vi "Main.vi"(8 "error in":errorcluster, 11 "Main UI in":refnum<class "Main UI.lvclass">) -> (0 "error out":errorcluster, 3 "Main UI out":refnum<class "Main UI.lvclass">)   [LabVIEW 2017, in "Main UI.lvclass"]
doc: "The <b>Queued Message Handler</b> of the Worker that owns this VI."
uses:
  Main UI.lvclass
  C:/Program Files (x86)/National Instruments/LabVIEW 2017/vi.lib/addons/_Workers/Library/Classes/Worker/Worker.lvclass
  Initialization Data.ctl
  Response Cases.ctl
  Main UI.lvclass/Main UI.ctl
  subPanel Worker/subPanel Worker.lvclass
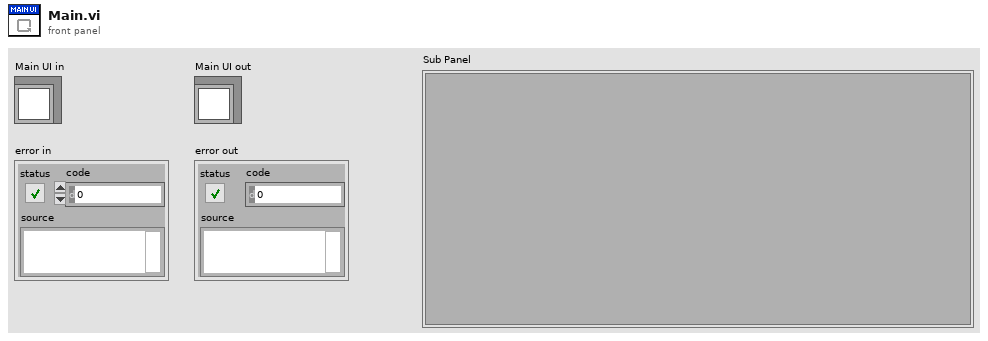
[diagram p1: front panel]
types:
  T1 = typedef "Main UI.lvclass/Initialization Data.ctl" = cluster{"Response Cases":T2}
  T2 = typedef "Main UI.lvclass/Response Cases.ctl" = cluster{"Placeholder - Can be deleted":string}
  T3 = typedef "subPanel Worker.lvclass/rwr_Get Main VI Ref Reply.ctl" = cluster{"VI Ref":refnum<vi>}
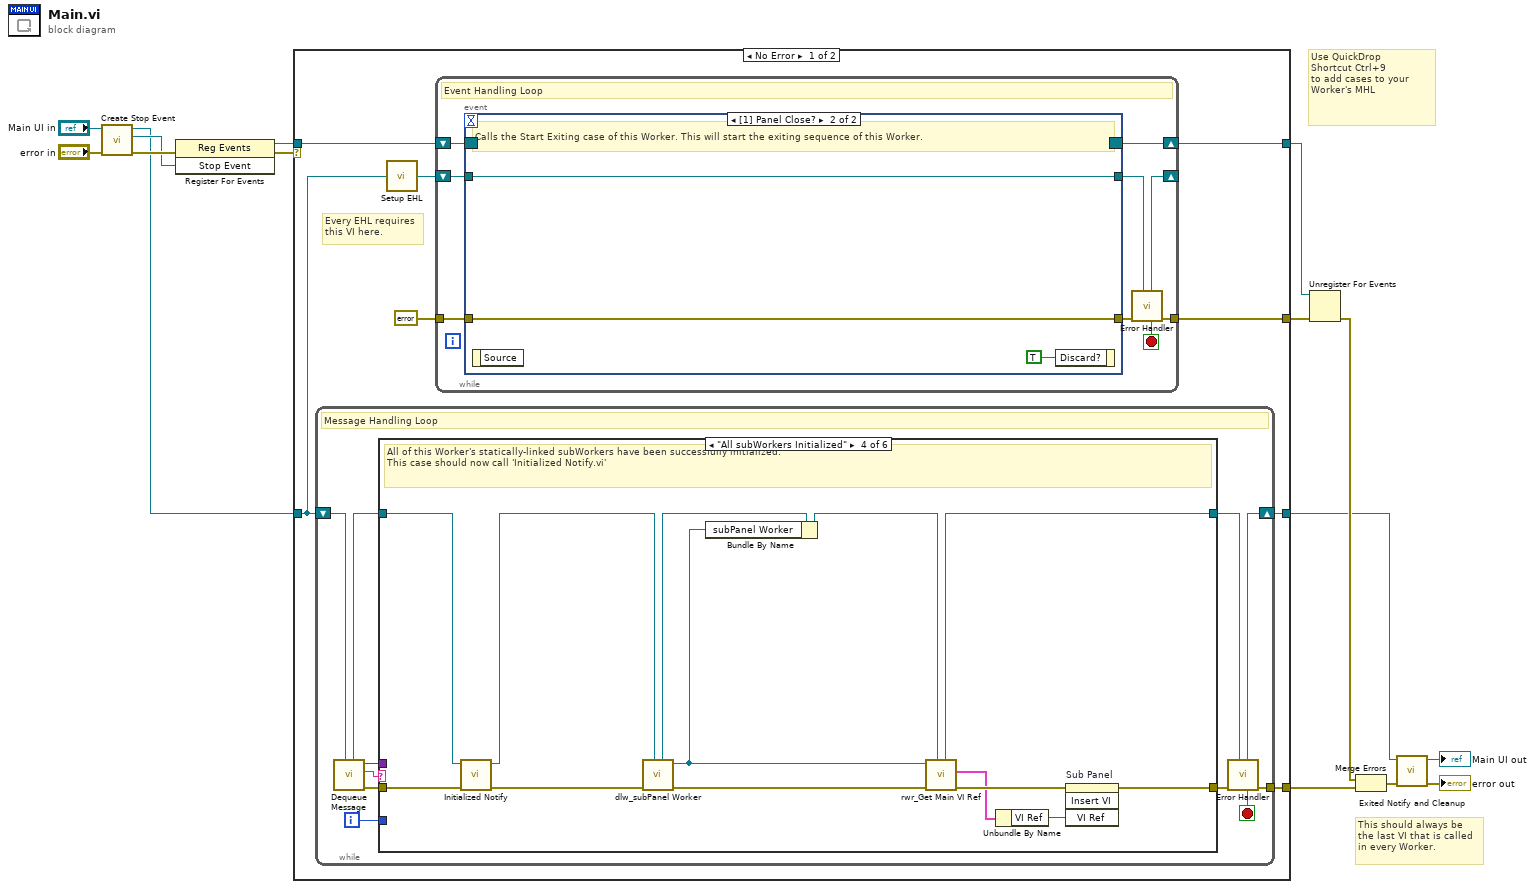
[diagram p0: block diagram]
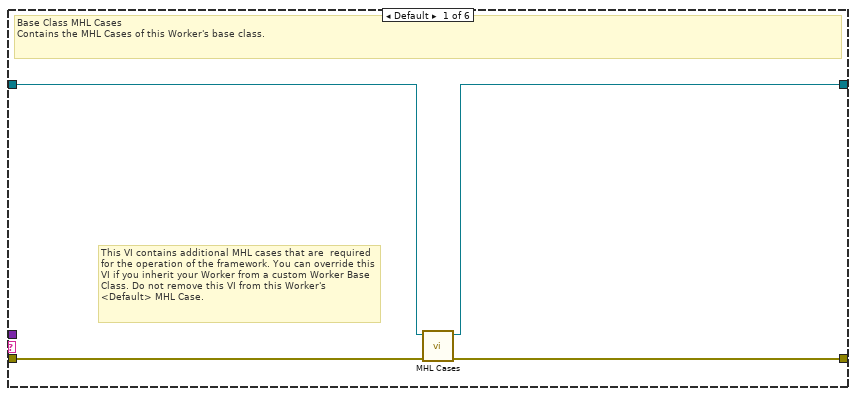
[diagram p2: hidden frame]
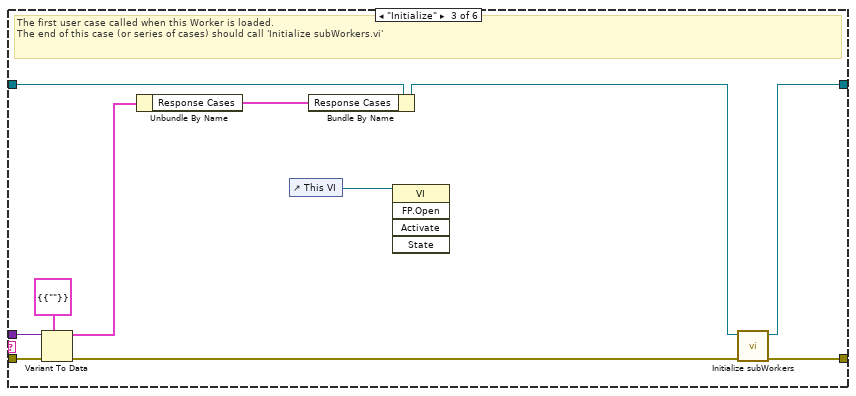
[diagram p4: hidden frame]
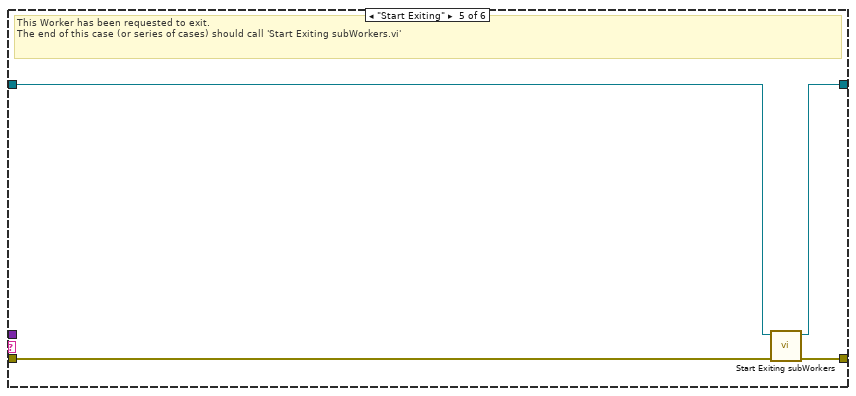
[diagram p5: hidden frame]
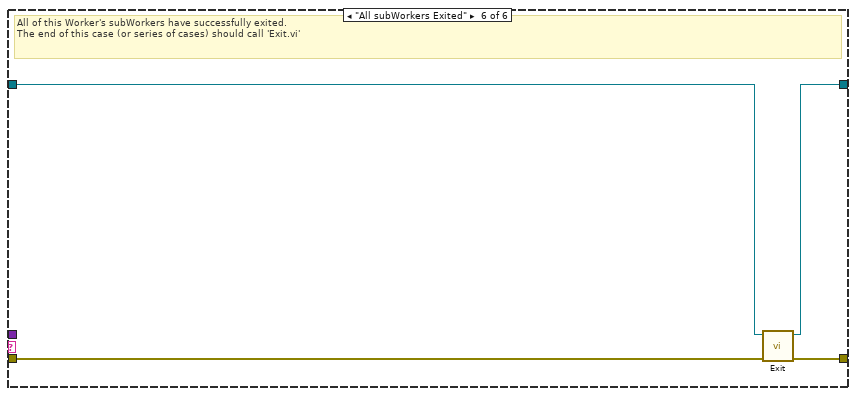
[diagram p6: hidden frame]
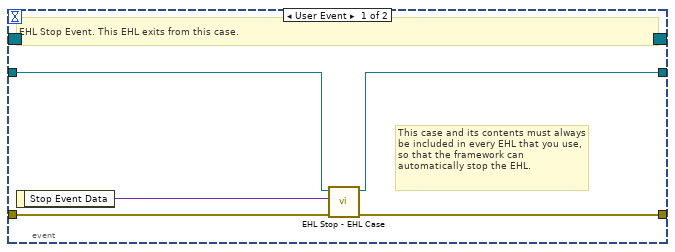
[diagram p7: hidden frame]
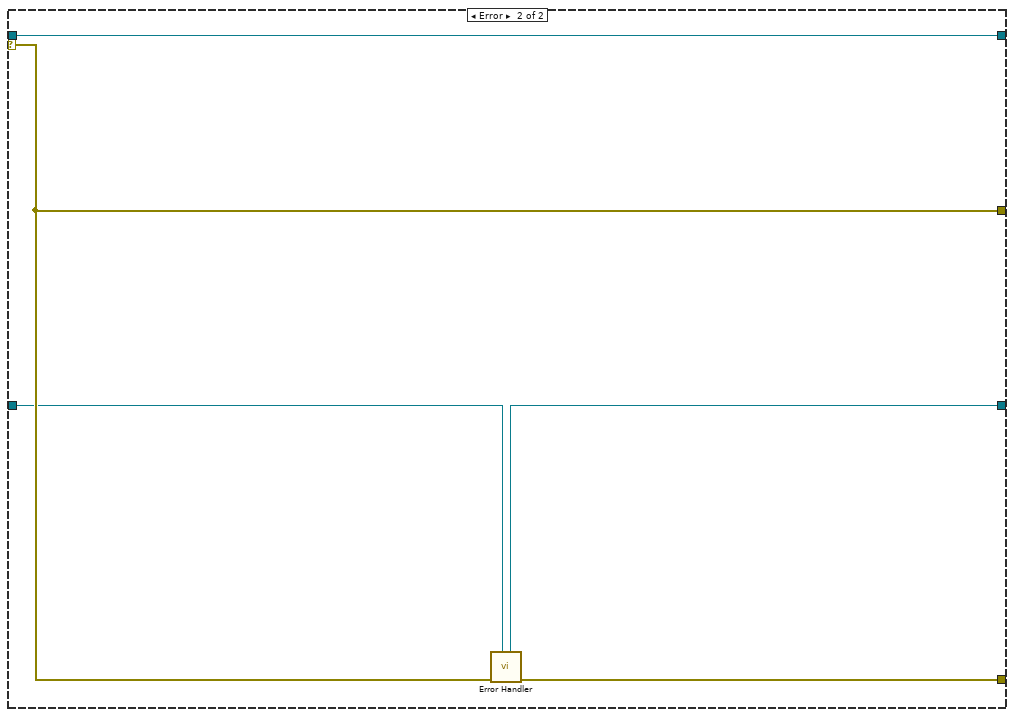
[diagram p8: hidden frame]
diagram:
  # "Use QuickDrop\nShortcut Ctrl+9\nto add cases to your\nWorker's MHL"
  # "This should always be the last VI that is called in every Worker."
  n1 = call-dynamic "Create Stop Event.vi"("error in"="error in", "Worker"="Main UI in") -> ("error out"=w10:errorcluster, "Stop Event"=w7:refnum<user-event>, "Worker out"=w4:refnum<class "Main UI.lvclass">)  [unwired: 7 in]
  n2 = register-events(error in=w10, w7) -> (reference out=w9:refnum<event-registration>, error out=w1:errorcluster)  [unwired: 1 in]
  n3 = case shown="No Error" w1 {
    tunnel: w4 -> [w18 w91]
    tunnel: [w16 w92] -> w8
    tunnel: w9 -> [w23 w93]
    tunnel: [w20 w94] -> w14
    tunnel: [w22 w93] -> w13
    tunnel: [w17 w90] -> w11
    selector: w1 -> [_ w94]
    frame No Error {
      # "Every EHL requires\nthis VI here."
      n4 = while {
        shift-right: [w32] -> w17
        shift-left: w18 -> [w34]
        tunnel: [w33] -> w16
        i -> [w24]
        stop <- w25 stop-if-true
        # "Message Handling Loop"
        n5 = call-dynamic "Dequeue Message.vi"("Worker"=w34) -> ("error out"=w31:errorcluster, "Case out"=w26:string, "Data out"=w27:variant, "Worker out"=w29:refnum<class "Main UI.lvclass">)  [unwired: 6 in, 1 out]
        n6 = case "Worker MHL Case Structure (DO NOT CHANGE LABEL NAME)" shown="\"All subWorkers Initialized\"" w26 {
          tunnel: w31 -> [w38 w39 w49 w63 w65 w72]
          tunnel: [w37 w39 w51 w55 w68 w71] -> w30
          tunnel: w29 -> [w36 w40 w48 w64 w66 w70]
          tunnel: [w35 w40 w50 w57 w67 w69] -> w28
          tunnel: w27 -> [_ _ w46 _ _ _]
          tunnel: w24 -> [_ _ _ _ _ _]
          frame Default {
            # "This VI contains additional MHL cases that are  required for the operation of the framework. You can override this VI if you inherit your Worker from a custom Worker Base Class. Do not remove this VI from this Worker's <Default> MHL Case."
            # "Base Class MHL Cases\nContains the MHL Cases of this Worker's base class."
            n7 = call-dynamic "MHL Cases.vi"("error in"=w38, "Worker in"=w36) -> ("error out"=w37:errorcluster, "Worker out"=w35:refnum<class "Main UI.lvclass">)  [unwired: 8 in]
          }
          frame "------------ FRAMEWORK CASES -----------" {
            # "Start of Workers Framework Cases"
          }
          frame "Initialize" {
            # "The first user case called when this Worker is loaded.\nThe end of this case (or series of cases) should call 'Initialize subWorkers.vi'"
            n8 = Variant To Data(error in=w49, type=T1 {"Response Cases"={"Placeholder - Can be deleted"=""}} ("Initialization Data"), Variant=w46) -> (data=w44:T1, error out=w47:errorcluster)
            n9 = Unbundle By Name(w44) -> ("Response Cases"=w43:T2)
            n10 = control-ref of="This VI"() -> (w41:refnum<vi>)
            n11 = Bundle By Name(cluster=w48, "Response Cases"=w43) -> (w45:refnum<class "Main UI.lvclass">)
            n12 = invoke class="VI" method="FP.Open"(reference=w41) -> ()  [unwired: 4 in, 5 out]
            n13 = call-dynamic "Initialize subWorkers.vi"("error in"=w47, "Worker"=w45) -> ("error out"=w51:errorcluster, "dup Worker out"=w50:refnum<class "Main UI.lvclass">)  [unwired: 8 in]
          }
          frame "All subWorkers Initialized" {
            # "All of this Worker's statically-linked subWorkers have been successfully initialized.\nThis case should now call 'Initialized Notify.vi'"
            n14 = call-dynamic "Initialized Notify.vi"("error in"=w63, "Worker"=w64) -> ("error out"=w62:errorcluster, "dup Worker out"=w60:refnum<class "Main UI.lvclass">)  [unwired: 8 in]
            n15 = call "dlw_subPanel Worker.vi"("Caller in"=w60, "error in"=w62) -> ("error out"=w61:errorcluster, "subPanel Worker out"=w52:refnum<class "subPanel Worker.lvclass">, "dup Caller out"=w59:refnum<class "Main UI.lvclass">)  [unwired: 7 in]
            n16 = Bundle By Name(cluster=w59, "subPanel Worker"=w52) -> (w58:refnum<class "Main UI.lvclass">)
            n17 = call "rwr_Get Main VI Ref.vi"("Caller in"=w58, "error in"=w61, "subPanel Worker in"=w52) -> ("error out"=w56:errorcluster, "Reply Data out"=w54:T3, "dup Caller out"=w57:refnum<class "Main UI.lvclass">)  [unwired: 5 in, 1 out]
            n18 = Unbundle By Name(w54) -> ("VI Ref"=w53:refnum<vi>)
            n19 = invoke on="Sub Panel" class="SubPnl" method="Insert VI"(error in=w56, "VI Ref"=w53) -> (error out=w55:errorcluster)  [unwired: 2 in, 3 out]
          }
          frame "Start Exiting" {
            # "This Worker has been requested to exit. \nThe end of this case (or series of cases) should call 'Start Exiting subWorkers.vi'"
            n20 = call-dynamic "Start Exiting subWorkers.vi"("error_in"=w65, "Worker"=w66) -> ("error out"=w68:errorcluster, "dup Worker out"=w67:refnum<class "Main UI.lvclass">)  [unwired: 8 in]
          }
          frame "All subWorkers Exited" {
            # "All of this Worker's subWorkers have successfully exited. \nThe end of this case (or series of cases) should call 'Exit.vi'"
            n21 = call-dynamic "Exit.vi"("error_in"=w72, "Worker"=w70) -> ("error out"=w71:errorcluster, "dup Worker out"=w69:refnum<class "Main UI.lvclass">)  [unwired: 8 in]
          }
        }
        n22 = call-dynamic "Error Handler.vi"("Worker"=w28, "error_in"=w30) -> ("error out"=w33:errorcluster, "Stop Loop"=w25:bool, "Worker out"=w32:refnum<class "Main UI.lvclass">)  [unwired: 7 in]
      }
      n23 = call-dynamic "Setup EHL.vi"("Worker"=w18) -> ("Worker out"=w19:refnum<class "Main UI.lvclass">)  [unwired: 14 in]
      n24 = while "Event Handling Loop" {
        shift-right: [w81] -> w22
        shift-left: w23 -> [w80]
        tunnel: [w76] -> w20
        tunnel: errorcluster {"status"=FALSE, "code"=0, "source"=""} ("error constant") -> [w78]
        shift-right: [w74] -> _
        shift-left: w19 -> [w79]
        stop <- w73 stop-if-true
        # "Event Handling Loop"
        n25 = event shown="[1] Panel Close?" {
          selector: w80 -> [_ _]
          dyn-events: [_ _] -> w81
          timeout: _ -> [_ _]
          tunnel: [w85 w88] -> w77
          tunnel: w78 -> [w86 w88]
          tunnel: w79 -> [w84 w87]
          tunnel: [w83 w87] -> w75
          event User Event {
            # "This case and its contents must always be included in every EHL that you use, so that the framework can automatically stop the EHL."
            # "EHL Stop Event. This EHL exits from this case."
            n26 = event-data() -> ("Stop Event Data"=w82:variant)  [unwired: 1 in]
            n27 = call-dynamic "EHL Stop - EHL Case.vi"("error in"=w86, "Stop Event Data"=w82, "Worker"=w84) -> ("error out"=w85:errorcluster, "Worker out"=w83:refnum<class "Main UI.lvclass">)  [unwired: 7 in]
          }
          event Panel Close? {
            # "Calls the Start Exiting case of this Worker. This will start the exiting sequence of this Worker."
            n28 = event-data() -> ()  [unwired: 1 in, 1 out]
            n29 = event-data("Discard?"=TRUE) -> ()  [unwired: 1 in, 1 out]
          }
        }
        n30 = call-dynamic "Error Handler.vi"("Worker"=w75, "error_in"=w77) -> ("error out"=w76:errorcluster, "Stop Loop"=w73:bool, "Worker out"=w74:refnum<class "Main UI.lvclass">)  [unwired: 7 in]
      }
    }
    frame Error {
      n31 = call-dynamic "Error Handler.vi"("Worker"=w91, "error_in"=w94) -> ("error out"=w92:errorcluster, "Worker out"=w90:refnum<class "Main UI.lvclass">)  [unwired: 7 in, 1 out]
    }
  }
  n32 = Unregister For Events(event registration refnum=w13, error in=w14) -> (error out=w15:errorcluster)
  n33 = Merge Errors(w15, w8) -> (w12:errorcluster)
  n34 = call-dynamic "Exited Notify and Cleanup.vi"("error_in"=w12, "Worker"=w11) -> ("error out"=→"error out":errorcluster, "dup Worker out"=→"Main UI out":refnum<class "Main UI.lvclass">)  [unwired: 8 in]
